vi "Actor Core.vi"(8 "error in":errorcluster, 11 "Data Viewer in":refnum<class "Data Viewer.lvclass">) -> (0 "error out":errorcluster, 3 "Actor out":refnum<class "Actor.lvclass">)   [LabVIEW 2017, in "2. Basic Panel Actors.lvlib" / "Data Viewer.lvclass"]
doc: "The user interface for this panel.\n----\nCopyright: MGI 2016\nAuthor: Derek Trepanier"
uses:
  Data Viewer.lvclass
  panel-actors/Source/Panel Actor/Panel Actor.lvclass
  D:/test/LabView_PanelManager/panel-actors/Source/Panel Actor/Panel Actor.lvclass
  <vilib>/ActorFramework/Actor/Actor.lvclass
panel:
  out "Waveform Graph":waveform(dbl)[](graph)
  # "Drag dataset(s) onto me"
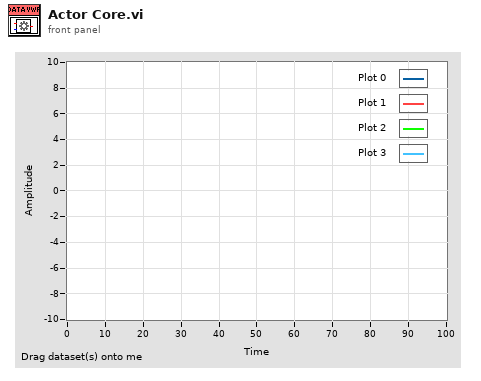
[diagram p1: front panel]
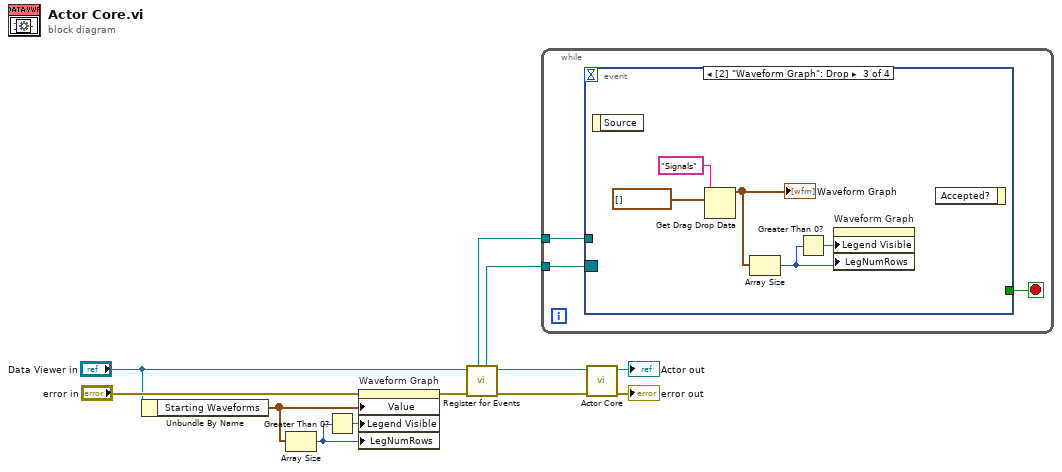
[diagram p0: block diagram]
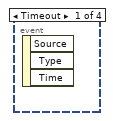
[diagram p2: hidden frame]
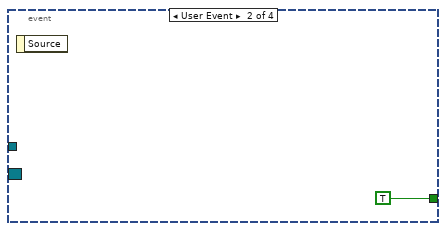
[diagram p3: hidden frame]
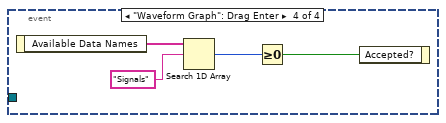
[diagram p4: hidden frame]
diagram:
  n1 = Unbundle By Name("Data Viewer in") -> ("Starting Waveforms"=w4:waveform(dbl)[])
  n2 = Array Size(array=w4) -> (size(s)=w2:i32)
  n3 = Greater Than 0?(x=w2) -> (x > 0?=w3:bool)
  n4 = property on="Waveform Graph" class="WFGraph (strict)"(error in="error in", "Value"=w4, "Legend Visible"=w3, "LegNumRows"=w2) -> (error out=w6:errorcluster)  [unwired: 1 in, 1 out]
  n5 = call "Register for Events.vi"("Error In"=w6, "Panel Actor in"="Data Viewer in") -> ("Error Out"=w10:errorcluster, "Panel Actor out"=w9:refnum<class "Data Viewer.lvclass">, "Pnl Actor"=w8:refnum<event-registration>, "Self Enqueuer"=w1:refnum<class "Message Enqueuer.lvclass">)  [unwired: 5 in, 1 out]
  n6 = while {
    tunnel: w8 -> [w15]
    tunnel: w1 -> [w13]
    stop <- w14 stop-if-true
    n7 = event shown="[2] \"Waveform Graph\": Drop" {
      selector: w15 -> [_ _ _ _]
      dyn-events: _ -> [_ _ _ _]
      timeout: _ -> [_ _ _ _]
      tunnel: [_ TRUE _ _] -> w14
      tunnel: w13 -> [_ _ _ _]
      event Timeout {
        n8 = event-data() -> ()  [unwired: 1 in, 3 out]
      }
      event User Event {
        n9 = event-data() -> ()  [unwired: 1 in, 1 out]
      }
      event "Waveform Graph": Drop {
        n10 = event-data() -> ()  [unwired: 1 in, 1 out]
        n11 = Get Drag Drop Data(8:waveform(dbl)[] [], 9:"Signals") -> (3:w17:waveform(dbl)[])  [unwired: 1 in, 1 out]
        "Waveform Graph" <- w17
        n12 = Array Size(array=w17) -> (size(s)=w19:i32)
        n13 = Greater Than 0?(x=w19) -> (x > 0?=w18:bool)
        n14 = property on="Waveform Graph" class="WFGraph (strict)"("Legend Visible"=w18, "LegNumRows"=w19) -> ()  [unwired: 2 in, 2 out]
        n15 = event-data() -> ()  [unwired: 2 in, 1 out]
      }
      event "Waveform Graph": Drag Enter {
        n16 = event-data() -> ("Available Data Names"=w25:string[])  [unwired: 1 in]
        n17 = Search 1D Array(1D array=w25, element="Signals") -> (index of element=w23:i32)  [unwired: 1 in]
        n18 = Greater Or Equal To 0?(x=w23) -> (x >= 0?=w22:bool)
        n19 = event-data("Accepted?"=w22) -> ()  [unwired: 1 in, 1 out]
      }
    }
  }
  n20 = call-parent "Actor Core.vi"("error in"=w10, "Panel Actor in"=w9) -> ("error out"=→"error out":errorcluster, "Actor out"=→"Actor out":refnum<class "Actor.lvclass">)  [unwired: 8 in]
